vi "Insert Sequence Call.vi"() -> ()   [LabVIEW 2016]
uses:
  TestStand API Tools/TSAT Engine Actions/TSAT Engine Actions.lvlib
  TestStand API Tools/Sequence File Actions/TSAT Sequence File Actions.lvlib
  TestStand API Tools/Sequence Actions/TSAT Sequence Actions.lvlib
  TestStand API Tools/Step Actions/TSAT Step Actions.lvlib
panel:
  out "error out":errorcluster
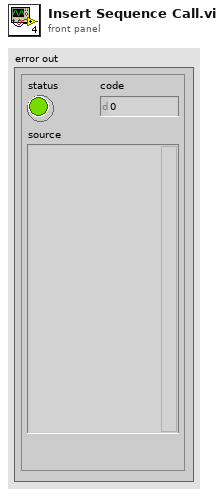
[diagram p1: front panel]
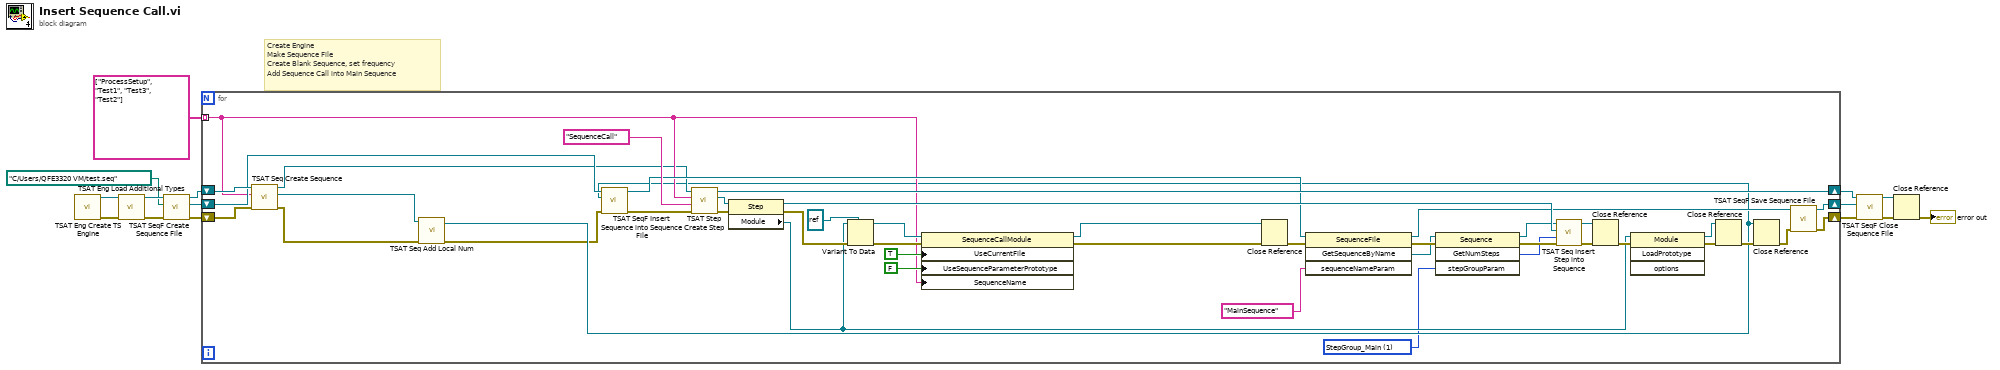
[diagram p0: block diagram]
diagram:
  # "Create Engine\nMake Sequence File\nCreate Blank Sequence, set frequency\nAdd Sequence Call into Main Sequence"
  n1 = call "TSAT Eng Create TS Engine.vi"() -> ("Error out"=w14:errorcluster, "Engine Reference"=w15:refnum<k7>)  [unwired: 10 in]
  n2 = call "TSAT Eng Load Additional Types.vi"("Error In"=w14, "Engine In"=w15) -> ("Error Out"=w13:errorcluster, "Engine Out"=w12:refnum<k7>)  [unwired: 8 in]
  n3 = call "TSAT SeqF Create Sequence File.vi"("Error In"=w13, "Sequence File Location"=path "C:/Users/QFE3320 VM/test.seq", "Engine In"=w12) -> ("Error Out"=w11:errorcluster, "Sequence File"=w2:refnum<k7>, "Engine Out"=w10:refnum<k7>)  [unwired: 6 in]
  n4 = for {
    tunnel: string[] ["ProcessSetup", "Test1", "Test3", "Test2"] -> [w26] mode=indexing
    shift-right: [w38] -> w7
    shift-left: w11 -> [w58]
    shift-right: [w36] -> w5
    shift-left: w10 -> [w57]
    shift-right: [w37] -> w6
    shift-left: w2 -> [w30]
    w16 = 1 items=["StepGroup_Setup", "StepGroup_Main", "StepGroup_Cleanup"] ("stepGroupParam")
    n5 = call "TSAT Seq Create Sequence.vi"("Error in"=w58, "Sequence Name"=w26, "Engine In"=w57) -> ("Error out"=w22:errorcluster, "Sequence Reference Out"=w24:refnum<k7>, "Engine Out"=w25:refnum<k7>)  [unwired: 6 in]
    n6 = call "TSAT Seq Add Local Num.vi"("Error In"=w22, "Sequence In"=w24) -> ("Error Out"=w21:errorcluster, "Sequence Out"=w23:refnum<k7>)  [unwired: 8 in]
    n7 = call "TSAT SeqF Insert Sequence into Sequence File.vi"("Error in"=w21, "Sequence to Insert"=w23, "Sequence File"=w30) -> ("Error Out"=w31:errorcluster, "Sequence File Out"=w29:refnum<k7>)  [unwired: 6 in, 1 out]
    n8 = call "TSAT Step Create Step.vi"("Error In"=w31, "stepTypeName"="SequenceCall", "Step Name"=w26, "Engine In"=w25) -> ("Error Out"=w53:errorcluster, "Step Reference"=w41:refnum<k7>, "Engine Out"=w36:refnum<k7>)  [unwired: 5 in]
    n9 = property class="Step"(reference=w41, error in=w53) -> (reference out=w40:refnum<k7>, error out=w42:errorcluster, "Module"=w33:refnum<k7>)
    n10 = Variant To Data(error in=w42, type=refnum<k7> refnum ("reference"), Variant=w33) -> (data=w52:refnum<k7>, error out=w51:errorcluster)
    n11 = property class="SequenceCallModule"(reference=w52, error in=w51, "UseCurrentFile"=TRUE, "UseSequenceParameterPrototype"=FALSE, "SequenceName"=w26) -> (reference out=w49:refnum<k7>, error out=w48:errorcluster)
    n12 = Close Reference(reference=w49, error in (no error)=w48) -> (error out=w47:errorcluster)
    n13 = invoke class="SequenceFile" method="GetSequenceByName"(reference=w29, error in=w47, "sequenceNameParam"="MainSequence") -> (reference out=w35:refnum<k7>, error out=w46:errorcluster, "GetSequenceByName"=w19:refnum<k7>)  [unwired: 1 in, 1 out]
    n14 = invoke class="Sequence" method="GetNumSteps"(reference=w19, error in=w46, "stepGroupParam"=w16) -> (reference out=w18:refnum<k7>, error out=w20:errorcluster, "GetNumSteps"=w17:i32)  [unwired: 1 in, 1 out]
    n15 = call "TSAT Seq Insert Step into Sequence.vi"("Error in"=w20, "Step Index"=w17, "Step to Add"=w40, "Sequence In"=w18) -> ("error out"=w45:errorcluster, "Sequence Out"=w44:refnum<k7>)  [unwired: 6 in]
    n16 = Close Reference(reference=w44, error in (no error)=w45) -> (error out=w43:errorcluster)
    n17 = invoke class="Module" method="LoadPrototype"(reference=w33, error in=w43) -> (reference out=w32:refnum<k7>, error out=w34:errorcluster)  [unwired: 2 in, 2 out]
    n18 = Close Reference(reference=w32, error in (no error)=w34) -> (error out=w39:errorcluster)
    n19 = Close Reference(reference=w23, error in (no error)=w39) -> (error out=w28:errorcluster)
    n20 = call "TSAT SeqF Save Sequence File.vi"("Error in"=w28, "Sequence File In"=w35) -> ("Error out"=w38:errorcluster, "Sequence File Out"=w37:refnum<k7>)  [unwired: 8 in]
  }
  n21 = call "TSAT SeqF Close Sequence File.vi"("Error In"=w7, "Sequence File In"=w6, "Engine In"=w5) -> ("Error Out"=w3:errorcluster, "Engine out"=w4:refnum<k7>)  [unwired: 7 in]
  n22 = Close Reference(reference=w4, error in (no error)=w3) -> (error out=→"error out":errorcluster)
